vi "NT Flush Data Updates.vi"(8 "error in (no error)":errorcluster) -> (0 "error out":errorcluster)   [LabVIEW 2017]
doc: "Flush any pending updates to connected Network Table and Smart Dashboard computers. Useful when you update a setpoint on a remote computer and want the robot to respond as quickly as possible.\n\nThis software is licensed. Open the labview\\readme\\WPI Robotics Library Open Source License.txt file for more information."
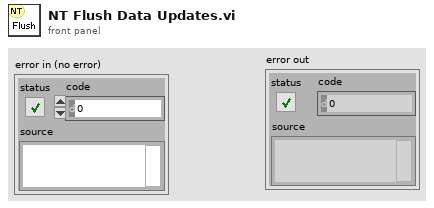
[diagram p1: front panel]
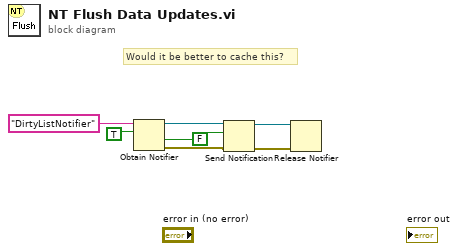
[diagram p0: block diagram]
diagram:
  w4 = FALSE ("IsClient")
  # "Would it be better to cache this?"
  n1 = Obtain Notifier(name (unnamed)="DirtyListNotifier", notification data type=TRUE ("IsClient"), create if not found? (T)=w4) -> (notifier out=w5:refnum<notifier>, error out=w3:errorcluster)  [unwired: 1 in, 1 out]
  n2 = Send Notification(notification=w4, notifier=w5, error in (no error)=w3) -> (notifier out=w2:refnum<notifier>, error out=w1:errorcluster)
  n3 = Release Notifier(notifier=w2, error in (no error)=w1) -> ()  [unwired: 1 in, 3 out]
